vi "SaveClusterToDiffTxt.vi"(3 "Save Cluster":T1 {"Select Layout" items=["Default"]}) -> (1 "DiffText":string)   [LabVIEW 2013]
uses:
  TypeDefs/SaveCluster.ctl
  VariableManagerCodes/VariableManager/VariableManager.lvclass
  DeviceVIs/Device/Device.lvclass
  <vilib>/Utility/miscctls.llb/LVStringsAndValuesArrayTypeDef_I32.ctl
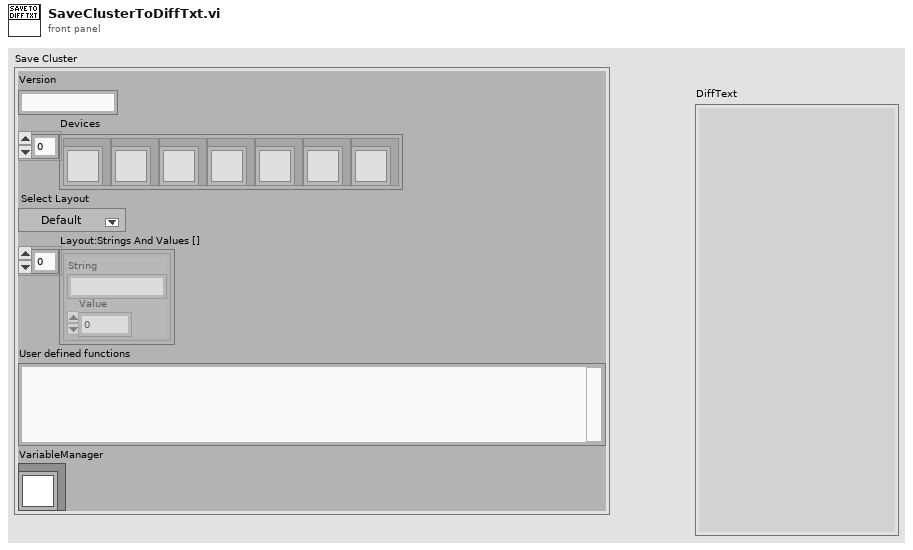
[diagram p1: front panel]
types:
  T1 = typedef "SaveCluster.ctl" = cluster{"Version":string, "Devices":refnum<class "Device.lvclass">[], "Select Layout":i32, "Layout:Strings And Values []":T2, "User defined functions":string, "VariableManager":refnum<class "VariableManager.lvclass">}
  T2 = typedef "LVStringsAndValuesArrayTypeDef_I32.ctl" = cluster{"String":string, "Value":i32}[]
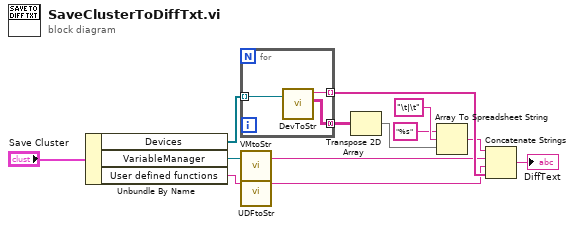
[diagram p0: block diagram]
diagram:
  n1 = Unbundle By Name("Save Cluster") -> ("Devices"=w11:refnum<class "Device.lvclass">[], "VariableManager"=w12:refnum<class "VariableManager.lvclass">, "User defined functions"=w13:string)
  n2 = for {
    tunnel: w11 -> [w16] mode=indexing
    tunnel: [w15] -> w4 mode=concatenating
    tunnel: [w14] -> w9 mode=indexing
    n3 = call "DevToStr.vi"("Device in"=w16) -> ("Device String"=w14:string, "Partial Table Transpose"=w15:string[][])  [unwired: 3 in]
  }
  n4 = call "VMtoStr.vi"("VariableManager in"=w12) -> ("VariablesString"=w2:string)  [unwired: 2 in]
  n5 = call "UDFtoStr.vi"("User Defined Functions"=w13) -> ("UDFString"=w3:string)  [unwired: 2 in]
  n6 = Transpose 2D Array(2D array=w4) -> (transposed array=w5:string[][])
  n7 = Array To Spreadsheet String(delimiter (Tab)="\t|\t", array=w5, 3:"%s" ("format string")) -> (spreadsheet string=w8:string)
  n8 = Concatenate Strings(w8, w2, w3, w9) -> (→"DiffText":string)
